vi "setApertureTime.vi"(8 "error in (no error)":errorcluster, 10 "Aperture Time [s]":dbl, 11 "DmmNiPxi in":refnum<class "DmmNi.lvclass">) -> (0 "error out":errorcluster, 3 "DmmNiPxi out":refnum<class "DmmNi.lvclass">)   [LabVIEW 2023, in "DmmNi.lvclass"]
doc: "<b>Author:</b> Wolfgang\n<b>Description:</b> Set Aperture Time in Seconds."
uses:
  DmmNi.lvclass
  DmmNi.lvclass/DmmNi.ctl
  Multimeter.lvclass
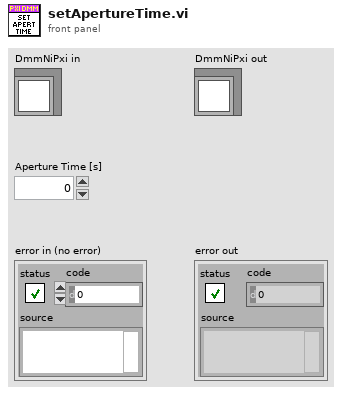
[diagram p1: front panel]
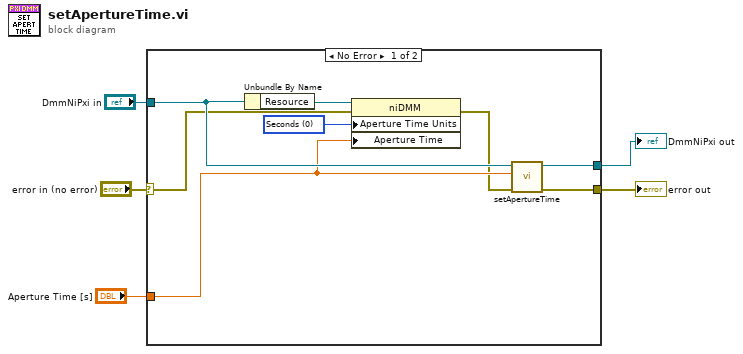
[diagram p0: block diagram]
diagram:
  n1 = case shown="No Error" "error in (no error)" {
    selector: "error in (no error)" -> [w7 w14]
    tunnel: [w13 w14] -> w5
    tunnel: [w12 w15] -> w4
    tunnel: "DmmNiPxi in" -> [w11 w15]
    tunnel: "Aperture Time [s]" -> [w8 _]
    frame No Error {
      w9 = 0 items=["Seconds", "Power Line Cycles"] ("Configuration:Advanced:Aperture Time Units")
      n2 = Unbundle By Name(w11) -> ("Resource"=w10:refnum<k15>)
      n3 = property class="niDMM"(reference=w10, error in=w7, "Aperture Time Units"=w9, "Aperture Time"=w8) -> (error out=w6:errorcluster)  [unwired: 1 out]
      n4 = call-parent "setApertureTime.vi"("error in (no error)"=w6, "Aperture Time [s]"=w8, "Multimeter in"=w11) -> ("error out"=w13:errorcluster, "Multimeter out"=w12:refnum<class "DmmNi.lvclass">)  [unwired: 7 in]
    }
    frame Error {
    }
  }
  "error out" <- w5
  "DmmNiPxi out" <- w4
